vi "DataSocket Read Connections Manager.vi"(7 "Action":enum16{"Get", "Close", "Close All"}(ring), 11 "URL":string) -> (0 "error out":errorcluster, 3 "connection id":refnum<k13>)   [LabVIEW 2024]
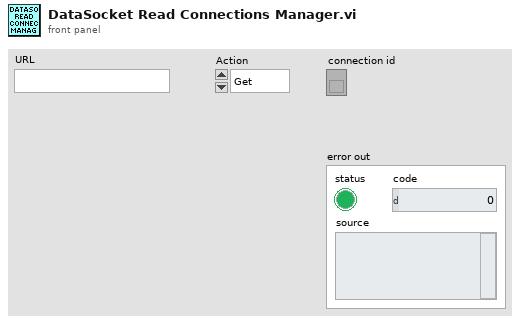
[diagram p1: front panel]
types:
  T1 = enum16{"Read", "Write", "ReadWrite", "BufferedRead", "BufferedReadWrite"}
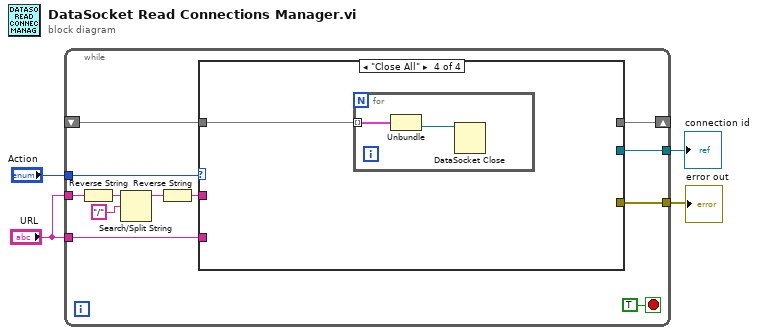
[diagram p0: block diagram]
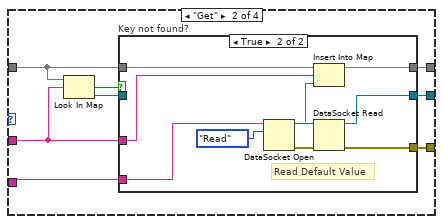
[diagram p3: hidden frame]
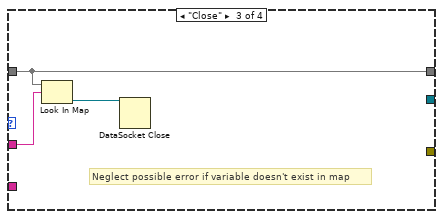
[diagram p5: hidden frame]
diagram:
  n1 = while {
    shift-right: [w14] -> _
    shift-left: _ -> [w13]
    tunnel: "URL" -> [w8]
    tunnel: [w12] -> w3
    tunnel: "Action" -> [w15]
    tunnel: "URL" -> [w6]
    tunnel: [w5] -> w1
    stop <- TRUE stop-if-true
    n2 = Reverse String(1:w8) -> (0:w11:string)
    n3 = Search/Split String(string=w11, search string/char (-)="/") -> (substring before match=w9:string)  [unwired: 1 in, 2 out]
    n4 = Reverse String(1:w9) -> (0:w7:string)
    n5 = case shown="\"Close All\"" w15 {
      tunnel: [_ w22 w36 _] -> w14
      tunnel: w13 -> [_ w23 w36 w39]
      tunnel: w7 -> [_ w21 w38 _]
      tunnel: [_ w19 _ _] -> w12
      tunnel: w6 -> [_ w18 _ _]
      tunnel: [_ w17 _ _] -> w5
      frame Default {
      }
      frame "Get" {
        n6 = Look In Map(map=w23, key=w21) -> (key not found?=w24:bool, value=w20:refnum<k13>)  [unwired: 1 in]
        n7 = case "Key not found?" shown="True" w24 {
          tunnel: w23 -> [w25 w35]
          tunnel: [w25 w34] -> w22
          tunnel: w21 -> [_ w28]
          tunnel: w20 -> [w26 _]
          tunnel: [w26 w31] -> w19
          tunnel: w18 -> [_ w29]
          tunnel: [_ w27] -> w17
          frame False {
          }
          frame True {
            # "Read Default Value"
            n8 = DataSocket Open(10:T1."Read" ("mode"), 11:w29) -> (0:w30:errorcluster, 3:w32:refnum<k13>)  [unwired: 2 in]
            n9 = DataSocket Read(8:w30, 11:w32) -> (0:w27:errorcluster, 3:w31:refnum<k13>)  [unwired: 3 in, 5 out]
            n10 = Insert Into Map(map in=w35, key=w28, value=w31) -> (map out=w34:map{string, refnum<k13>})  [unwired: 2 out]
          }
        }
      }
      frame "Close" {
        # "Neglect possible error if variable doesn't exist in map"
        n11 = Look In Map(map=w36, key=w38) -> (value=w37:refnum<k13>)  [unwired: 1 in, 1 out]
        n12 = DataSocket Close(11:w37) -> ()  [unwired: 2 in, 2 out]
      }
      frame "Close All" {
        n13 = for {
          tunnel: w39 -> [w41] mode=indexing
          n14 = Unbundle(w41) -> ("connection id"=w40:refnum<k13>)  [unwired: 1 out]
          n15 = DataSocket Close(11:w40) -> ()  [unwired: 2 in, 2 out]
        }
      }
    }
  }
  "connection id" <- w3
  "error out" <- w1
